vi "Set Type.vi"(10 "Type":refnum<class "Type.lvclass">, 11 "IntegerPanel in":refnum<class "IntegerPanel.lvclass">) -> (3 "IntegerPanel out":refnum<class "IntegerPanel.lvclass">)   [LabVIEW 2020, in "Conditum-Tools.lvlib" / "IntegerPanel.lvclass"]
uses:
  IntegerPanel.lvclass
  Conditum-Clone/Columns/Type/Type.lvclass
  IntegerPanel.lvclass/IntegerPanel.ctl
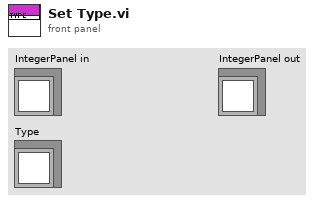
[diagram p1: front panel]
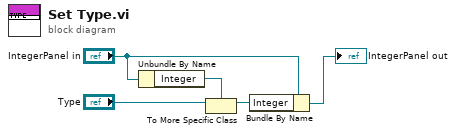
[diagram p0: block diagram]
diagram:
  n1 = Unbundle By Name("IntegerPanel in") -> ("Integer"=w4:refnum<class "Integer.lvclass">)
  n2 = To More Specific Class(target class=w4, reference="Type") -> (specific class reference=w5:refnum<class "Integer.lvclass">)  [unwired: 1 in, 1 out]
  n3 = Bundle By Name(cluster="IntegerPanel in", "Integer"=w5) -> (→"IntegerPanel out":refnum<class "IntegerPanel.lvclass">)
